vi "TrajectoryTrend.vi"() -> ()   [LabVIEW 2025]
uses:
  <vilib>/Rock Robotics/Network Tables/NT Read Number.vi
  <vilib>/Rock Robotics/Network Tables/NT Read Boolean.vi
panel:
  out "Trajectory Chart":T1(graph)
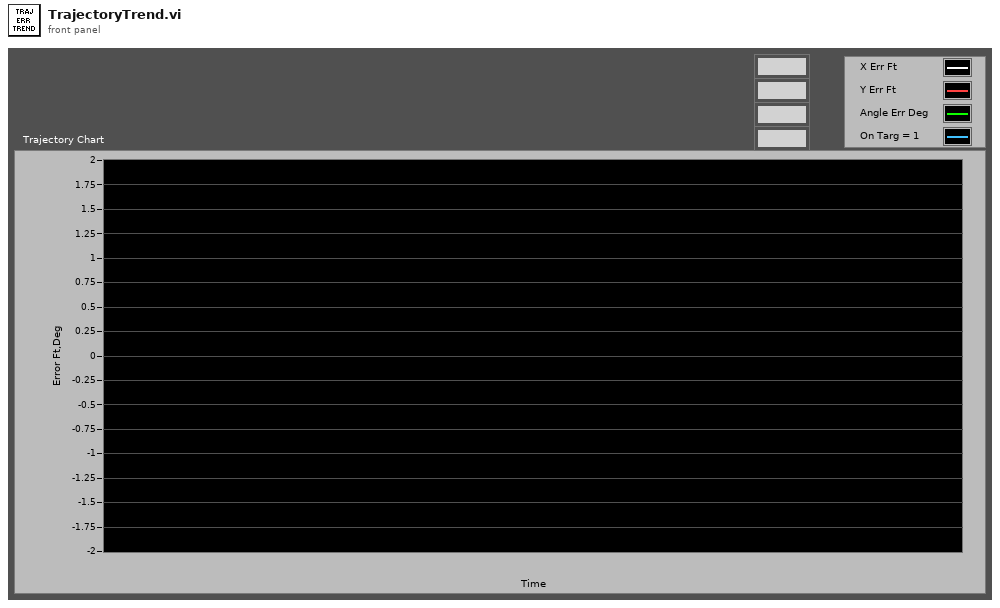
[diagram p1: front panel]
types:
  T1 = cluster{"value":dbl, "value":dbl, "value":dbl, dbl}
  T2 = enum8{"Tele-Op Disabled", "Tele-Op Enabled", "Auto Disabled", "Auto Enabled", "Test Disabled", "Test Enabled", "Disconnected", "No Code", "E-Stop"}
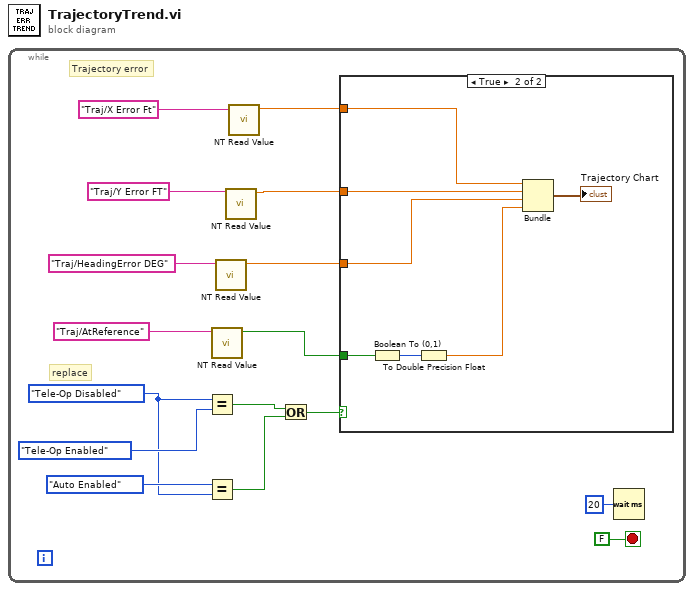
[diagram p0: block diagram]
diagram:
  n1 = while {
    stop <- FALSE stop-if-true
    w1 = T2."Tele-Op Disabled" ("x")
    # "replace"
    # "Trajectory error"
    n2 = Equal?(x=w1, y=T2."Tele-Op Enabled") -> (x = y?=w12:bool)
    n3 = Equal?(x=T2."Auto Enabled" ("y"), y=w1) -> (x = y?=w11:bool)
    n4 = call-poly <vilib>:"NT Read Value.vi"("name"="Traj/AtReference" ("Name")) -> ("value"=w8:bool)  [unwired: 8 in, 2 out]
    n5 = call-poly <vilib>:"NT Read Value.vi"("name"="Traj/HeadingError DEG" ("Name")) -> ("value"=w6:dbl)  [unwired: 8 in, 2 out]
    n6 = call-poly <vilib>:"NT Read Value.vi"("name"="Traj/Y Error FT" ("Name")) -> ("value"=w4:dbl)  [unwired: 8 in, 2 out]
    n7 = call-poly <vilib>:"NT Read Value.vi"("name"="Traj/X Error Ft" ("Name")) -> ("value"=w2:dbl)  [unwired: 8 in, 2 out]
    n8 = Or(x=w12, y=w11) -> (x .or. y?=w10:bool)
    n9 = case shown="True" w10 {
      tunnel: w8 -> [_ w19]
      tunnel: w6 -> [_ w23]
      tunnel: w4 -> [_ w22]
      tunnel: w2 -> [_ w20]
      frame False {
      }
      frame True {
        n10 = Boolean To (0,1)(Boolean=w19) -> (0, 1=w18:i16)
        n11 = To Double Precision Float(number=w18) -> (double precision float=w17:dbl)
        n12 = Bundle("value"=w20, "value"=w22, "value"=w23, w17) -> (→"Trajectory Chart":T1)  [unwired: 1 in]
      }
    }
    n13 = Wait (ms)(milliseconds to wait=u32 20) -> ()  [unwired: 1 out]
  }
